vi "SaveLogCounterToFile.vi"(11 "number":i32) -> ()   [LabVIEW 2013]
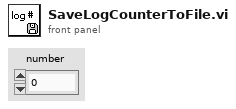
[diagram p1: front panel]
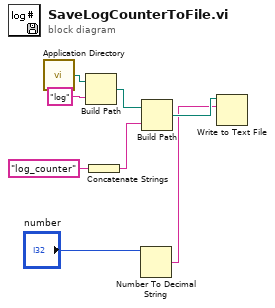
[diagram p0: block diagram]
diagram:
  n1 = call <vilib>:"Application Directory.vi"() -> ("Application Directory"=w8:path)
  n2 = Build Path(base path=w8, name or relative path="log") -> (appended path=w6:path)
  n3 = Concatenate Strings("log_counter" ("string")) -> (w4:string)
  n4 = Number To Decimal String(number="number") -> (decimal integer string=w2:string)  [unwired: 1 in]
  n5 = Build Path(base path=w6, name or relative path=w4) -> (appended path=w3:path)
  n6 = Write to Text File(file (use dialog)=w3, text=w2) -> ()  [unwired: 2 in, 3 out]
